vi "Get NiDAQmx SetChanAttributeString Request.vi"(8 "error in (no error)":errorcluster, 11 "gRPCid":T1) -> (0 "error out":errorcluster, 2 "Message Data":T2, 3 "gRPCid out":T1)   [LabVIEW 2021, in "NI DAQmx_server.lvlib" / "NiDAQmx.lvclass"]
uses:
  NiDAQmx.lvclass
  <vilib>/gRPC/LabVIEW gRPC Library/Shared/grpcId.ctl
  NiDAQmx.lvclass/NiDAQmx.ctl
  NI DAQmx_server.lvlib
  <vilib>/gRPC/LabVIEW gRPC Library/grpc-lvsupport-release.lvlib
  RPC Messages/nidevice_grpc_Session_session/nidevice_grpc_Session_session.lvclass
  RPC Messages/nidevice_grpc_Session.ctl
  RPC Messages/nidaqmx_grpc_SetChanAttributeStringRequest_attribute_enum/nidaqmx_grpc_SetChanAttributeStringRequest_attribute_enum.lvclass
  RPC Messages/nidaqmx_grpc_SetChanAttributeStringRequest.ctl
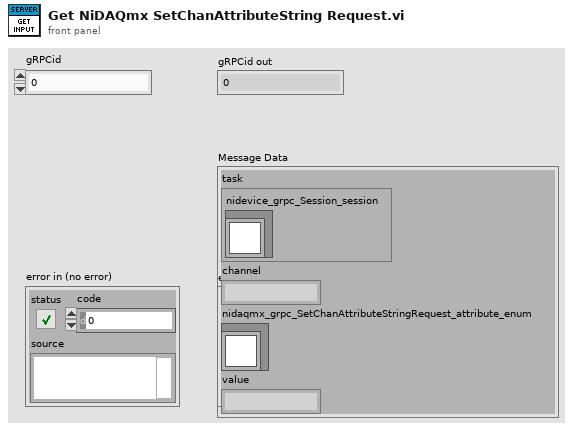
[diagram p1: front panel]
types:
  T1 = typedef "grpc-lvsupport-release.lvlib/grpcId.ctl" = u64
  T2 = typedef "NI DAQmx_server.lvlib/nidaqmx_grpc_SetChanAttributeStringRequest.ctl" = cluster{"task":T3, "channel":string, "nidaqmx_grpc_SetChanAttributeStringRequest_attribute_enum":refnum<class "nidaqmx_grpc_SetChanAttributeStringRequest_attribute_enum.lvclass">, "value":string}
  T3 = typedef "NI DAQmx_server.lvlib/nidevice_grpc_Session.ctl" = cluster{"nidevice_grpc_Session_session":refnum<class "nidevice_grpc_Session_session.lvclass">}
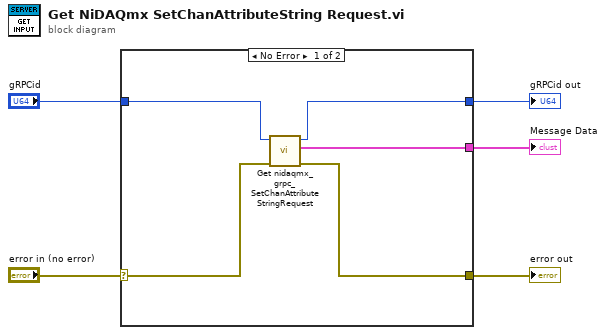
[diagram p0: block diagram]
diagram:
  n1 = case shown="No Error" "error in (no error)" {
    selector: "error in (no error)" -> [w10 w12]
    tunnel: [w9 w12] -> w4
    tunnel: [w8 _] -> w3
    tunnel: "gRPCid" -> [w7 w11]
    tunnel: [w6 w11] -> w1
    frame No Error {
      n2 = call "Get nidaqmx_grpc_SetChanAttributeStringRequest.vi"("error in (no error)"=w10, "gRPCid"=w7) -> ("error out"=w9:errorcluster, "package_templatemessage"=w8:T2, "gRPCid out"=w6:T1)  [unwired: 7 in]
    }
    frame Error {
    }
  }
  "error out" <- w4
  "Message Data" <- w3
  "gRPCid out" <- w1
